vi "ma_manage resamp timing continuous.vi"(0 "waveform in":waveform(dbl), 5 "dt":dbl=1.0 format="%.2p", 7 "state info in":cluster{"buffer":dbl[], "t0 history":timestamp} {"t0 history" format="%<%.4X>T"; "buffer" format="%.2p"}, 11 "error in":errorcluster, 12 "filter half-length (s)":dbl=1.0 format="%.2p") -> (4 "waveform to be processed":waveform(dbl), 6 "#elements":i32, 8 "state info out":cluster{"buffer":dbl[], "t0 history":timestamp} {"t0 history" format="%<%.4X>T"; "buffer" format="%.2p"}, 10 "used t0":timestamp format="%<%.4X>T", 14 "t0 adjusted warning":bool, 15 "error out":errorcluster)   [LabVIEW 2020, in "NI_MAPro.lvlib"]
doc: "This VI re-samples an unevenly sampled input signal to an evenly sampled waveform according to specified t0 and dt. If the specified t0 value is less than the first value of input X-array (that is the timestamp of the first input sample), then the VI will coerce t0 to the first valid value (greater than X(0)) that also fulfill the relation:\n\nT0_adjusted - t0_in = n * dt_in\n\nThis guarranty that any later comparison of waveforms will be correct with repsect to absolute time."
uses:
  NI_MAPro.lvlib
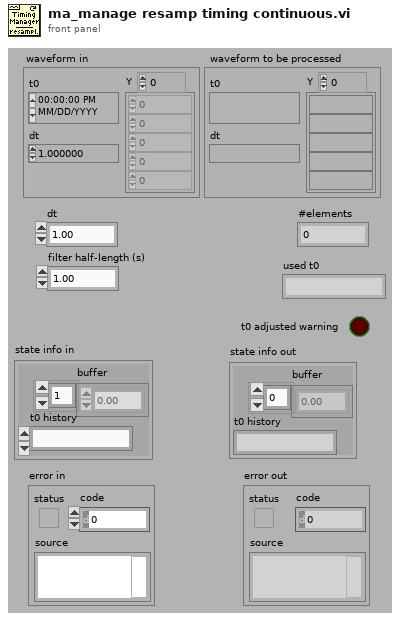
[diagram p1: front panel]
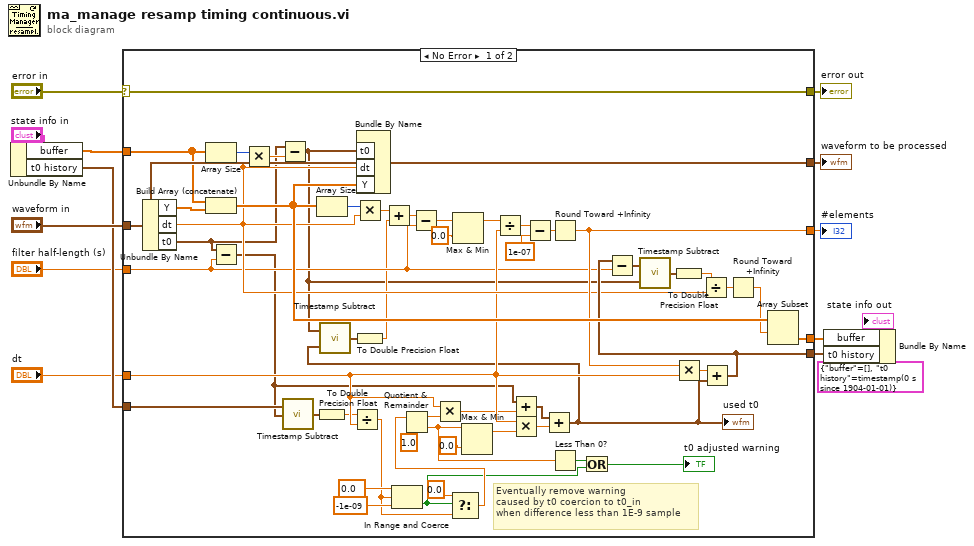
[diagram p0: block diagram]
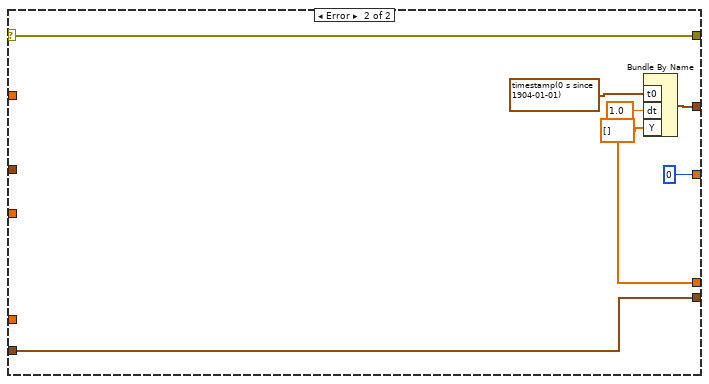
[diagram p2: hidden frame]
diagram:
  n1 = Unbundle By Name("state info in") -> ("buffer"=w7:dbl[], "t0 history"=w8:timestamp)
  n2 = case shown="No Error" "error in" {
    selector: "error in" -> [w29 w75]
    tunnel: [w29 w75] -> w13
    tunnel: "waveform in" -> [w64 _]
    tunnel: w8 -> [w63 w74]
    tunnel: "dt" -> [w31 _]
    tunnel: [w49 w74] -> w14
    tunnel: [w60 w73] -> w11
    tunnel: [w50 0] -> w10
    tunnel: w7 -> [w56 _]
    tunnel: "filter half-length (s)" -> [w30 _]
    tunnel: [w52 w70] -> w4
    frame No Error {
      # "Eventually remove warning\ncaused by t0 coercion to t0_in\nwhen difference less than 1E-9 sample"
      n3 = Unbundle By Name(w64) -> ("Y"=w57:dbl[], "dt"=w46:dbl, "t0"=w28:timestamp)
      n4 = Array Size(array=w56) -> (size(s)=w62:i32)
      n5 = Build Array (concatenate)(w56, w57) -> (w53:dbl[])
      n6 = Subtract(x=w28, y=w30) -> (x-y=w24:timestamp)
      n7 = Multiply(x=w62, y=w46) -> (x*y=w61:dbl)
      n8 = Subtract(x=w28, y=w61) -> (x-y=w16:timestamp)
      n9 = call "Timestamp Subtract.vi"("y"=w24, "x"=w63) -> ("x - y"=w22:timestamp)
      n10 = Array Size(array=w53) -> (size(s)=w44:i32)
      n11 = To Double Precision Float(number=w22) -> (double precision float=w23:dbl)
      n12 = Divide(x=w23, y=w31) -> (x/y=w36:dbl)
      n13 = Multiply(x=w44, y=w46) -> (x*y=w54:dbl)
      n14 = Bundle By Name(cluster=w64, "t0"=w16, "dt"=w46, "Y"=w53) -> (w60:waveform(dbl))
      n15 = In Range and Coerce(upper limit=0.0, x=w36, lower limit=-1e-09) -> (In Range?=w33:bool)  [unwired: 1 out]
      n16 = Select(t=0.0, s=w33, f=w36) -> (s? t:f=w35:dbl)
      n17 = Quotient & Remainder(x=w35, y=1.0) -> (x-y*floor(x/y)=w40:dbl, floor(x/y)=w65:dbl)
      n18 = Multiply(x=w31, y=w40) -> (x*y=w25:dbl)
      n19 = Max & Min(x=w65, y=0.0) -> (max(x,y)=w67:dbl)  [unwired: 1 out]
      n20 = Add(x=w24, y=w25) -> (x+y=w27:timestamp)
      n21 = Multiply(x=w31, y=w67) -> (x*y=w26:dbl)
      n22 = Add(x=w27, y=w26) -> (x+y=w20:timestamp)
      "used t0" <- w20
      n23 = call "Timestamp Subtract.vi"("y"=w20, "x"=w16) -> ("x - y"=w21:timestamp)
      n24 = To Double Precision Float(number=w21) -> (double precision float=w19:dbl)
      n25 = Add(x=w54, y=w19) -> (x+y=w55:dbl)
      n26 = Subtract(x=w55, y=w30) -> (x-y=w45:dbl)
      n27 = Max & Min(x=w45, y=0.0) -> (max(x,y)=w58:dbl)  [unwired: 1 out]
      n28 = Divide(x=w58, y=w31) -> (x/y=w42:dbl)
      n29 = Subtract(x=w42, y=1e-07) -> (x-y=w41:dbl)
      n30 = Round Toward +Infinity(x=w41) -> (ceil(x): smallest int >= x=w50:dbl)
      n31 = Less Than 0?(x=w65) -> (x < 0?=w34:bool)
      n32 = Or(x=w34, y=w33) -> (x .or. y?=→"t0 adjusted warning":bool)
      n33 = Multiply(x=w50, y=w31) -> (x*y=w51:dbl)
      n34 = Add(x=w51, y=w20) -> (x+y=w49:timestamp)
      n35 = Subtract(x=w49, y=w30) -> (x-y=w17:timestamp)
      n36 = call "Timestamp Subtract.vi"("y"=w16, "x"=w17) -> ("x - y"=w18:timestamp)
      n37 = To Double Precision Float(number=w18) -> (double precision float=w15:dbl)
      n38 = Divide(x=w15, y=w46) -> (x/y=w48:dbl)
      n39 = Round Toward +Infinity(x=w48) -> (ceil(x): smallest int >= x=w47:dbl)
      n40 = Array Subset(array=w53, index=w47) -> (w52:dbl[])  [unwired: 1 in]
    }
    frame Error {
      w70 = dbl[] [] ("Y")
      n41 = Bundle By Name("t0"=timestamp(0 s since 1904-01-01), "dt"=1.0, "Y"=w70) -> (w73:waveform(dbl))  [unwired: 1 in]
    }
  }
  "error out" <- w13
  "waveform to be processed" <- w11
  "#elements" <- w10
  n42 = Bundle By Name(cluster=cluster{"buffer":dbl[], "t0 history":timestamp} {"buffer"=[], "t0 history"=timestamp(0 s since 1904-01-01)} ("state info out"), "buffer"=w4, "t0 history"=w14) -> (→"state info out":cluster{"buffer":dbl[], "t0 history":timestamp})
